vi "VA_ImgRecog.vi"(0 "Image":T1, 1 "Template":T1) -> (2 "Image Dst Out":T1, 3 "X":sgl, 4 "Y":sgl, 5 "Degrees":dbl)   [LabVIEW 2009]
uses:
  <vilib>/vision/Image Controls.llb/IMAQ Image.ctl
  <vilib>/vision/NI_Vision_Development_Module.lvlib
panel:
  in  "ROIC":T2
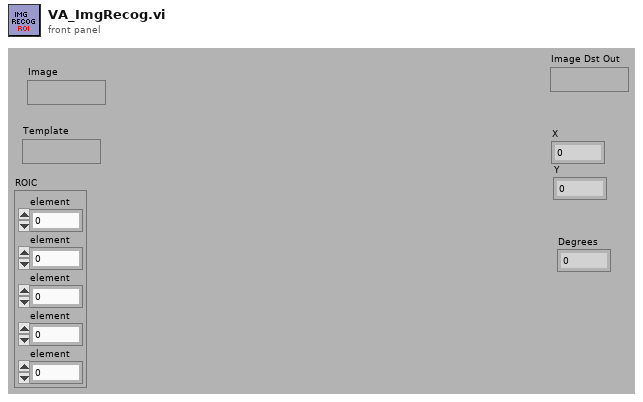
[diagram p1: front panel]
types:
  T1 = typedef "IMAQ Image.ctl" = refnum<image>
  T2 = cluster{"element":dbl, "element":dbl, "element":dbl, "element":dbl, "element":dbl}
  T3 = cluster{"Match Mode":u16, "Minimum Match Score":sgl, "SubPixel Accuracy":bool, "Rotation Angle Ranges":cluster{"Start":sgl, "End":sgl}[], "Show Search Area":bool, "Show Feature Found":bool, "Show Result":bool}
  T4 = cluster{"Point1":cluster{"X":sgl, "Y":sgl}, "Point2":cluster{"X":sgl, "Y":sgl}}
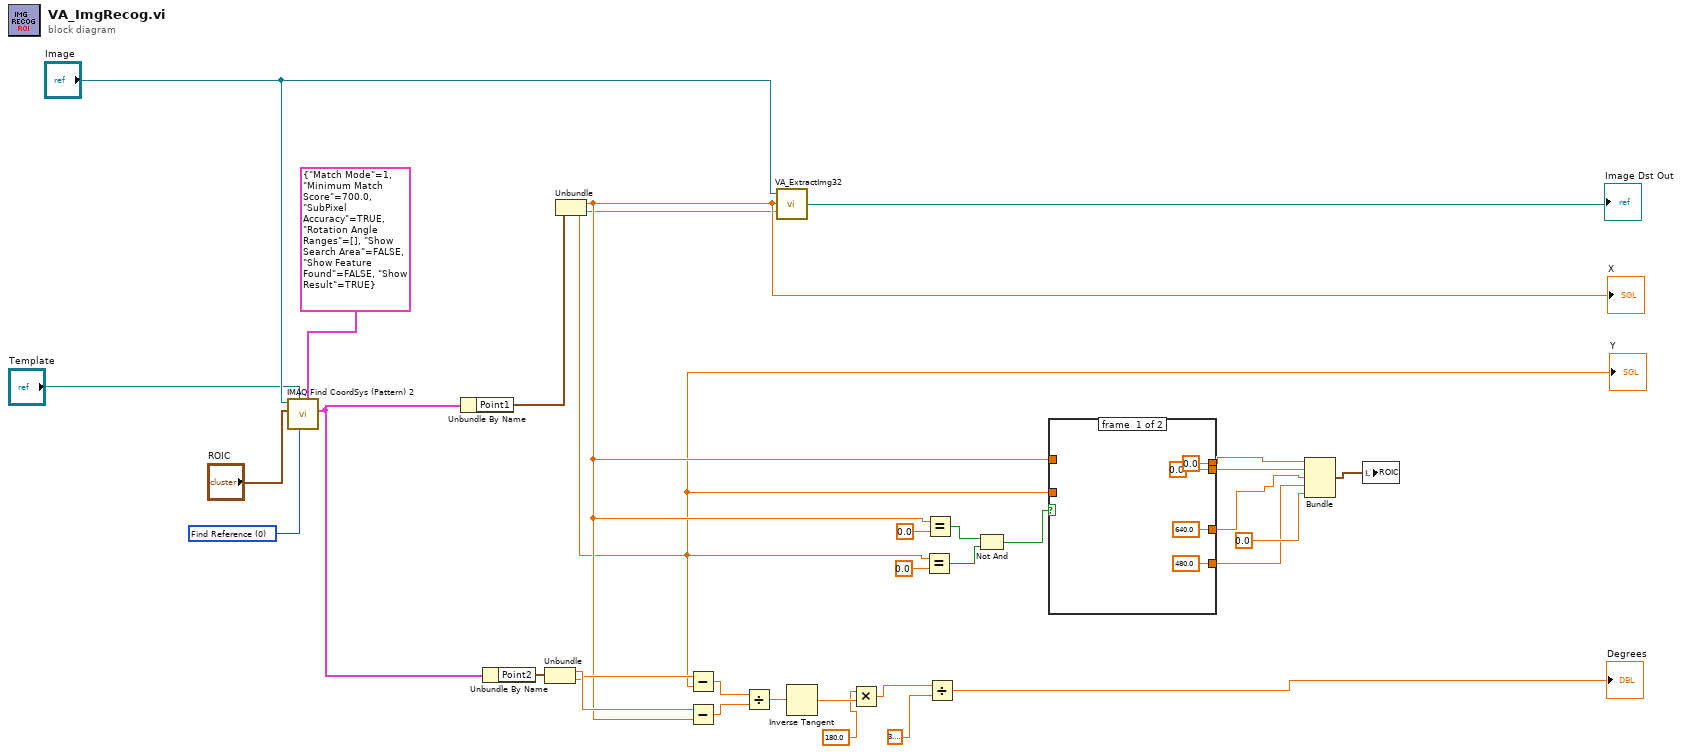
[diagram p0: block diagram]
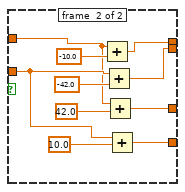
[diagram p2: hidden frame]
diagram:
  w32 = u16 0 items=["Find Reference", "Update CoordSys"] ("Function")
  n1 = call "IMAQ Find CoordSys (Pattern) 2"("Settings"=T3 {"Match Mode"=1, "Minimum Match Score"=700.0, "SubPixel Accuracy"=TRUE, "Rotation Angle Ranges"=[], "Show Search Area"=FALSE, "Show Feature Found"=FALSE, "Show Result"=TRUE}, "Mode"=w32, "Template"="Template", "Search Rect"="ROIC", "Image"="Image") -> ("Main Axis"=w28:T4)  [unwired: 2 in, 4 out]
  n2 = Unbundle By Name(w28) -> ("Point1"=w30:cluster{"X":sgl, "Y":sgl})
  n3 = Unbundle By Name(w28) -> ("Point2"=w29:cluster{"X":sgl, "Y":sgl})
  n4 = Unbundle(w29) -> ("X"=w20:sgl, "Y"=w19:sgl)
  n5 = Unbundle(w30) -> ("X"=w4:sgl, "Y"=w3:sgl)
  "X" <- w4
  "Y" <- w3
  n6 = Subtract(x=w19, y=w3) -> (x-y=w27:sgl)
  n7 = Subtract(x=w20, y=w4) -> (x-y=w26:sgl)
  n8 = Divide(x=w27, y=w26) -> (x/y=w25:sgl)
  n9 = call "VA_ExtractImg32.vi"("y"=w3, "x"=w4, "Image Src"="Image") -> ("Image Dst Out"=→"Image Dst Out":T1)
  n10 = Inverse Tangent(1:w25) -> (0:w24:sgl)
  n11 = Multiply(x=sgl 180.0, y=w24) -> (x*y=w22:sgl)
  n12 = Equal?(x=w3, y=sgl 0.0) -> (x = y?=w7:bool)
  n13 = Equal?(x=w4, y=sgl 0.0) -> (x = y?=w8:bool)
  n14 = Divide(x=w22, y=3.141592653589793) -> (x/y=→"Degrees":dbl)
  n15 = Not And(1:w7, 2:w8) -> (0:w6:bool)
  n16 = case shown="True" w6 {
    tunnel: [sgl 0.0 w42] -> w15
    tunnel: [sgl 0.0 w41] -> w14
    tunnel: [sgl 640.0 w40] -> w13
    tunnel: [sgl 480.0 w39] -> w12
    tunnel: w3 -> [_ w38]
    tunnel: w4 -> [_ w37]
    frame #0 {
    }
    frame #1 {
      n17 = Add(x=w37, y=sgl -10.0) -> (x+y=w42:sgl)
      n18 = Add(x=w38, y=sgl -42.0) -> (x+y=w41:sgl)
      n19 = Add(x=w37, y=sgl 42.0) -> (x+y=w40:sgl)
      n20 = Add(x=w38, y=sgl 10.0) -> (x+y=w39:sgl)
    }
  }
  n21 = Bundle(w15, w14, w13, w12, "element"=0.0) -> (w16:cluster{sgl, sgl, sgl, sgl, "element":dbl})  [unwired: 1 in]
  n22 = local write "ROIC"(w16) -> ()
